vi "send_scenario_config.vi"(0 "simx in":T1={"Config"={"Trajectory"={"Number of frames"=0, "Frame number"=0, "Trajectory"=""}, "Weather"={"id"=""}}, "Connections"={"Simulator Connection"=refnum, "server_ip"="127.0.0.1", "Port"=0, "Sensor connections"=[]}, "Map"={"lanes"={"x"=[], "y"=[], "z"=[]}, "StartPosition"={"start_points"={"locations"=[], "rotations"=[], "type"=[]}, "StartRotation"=[], "StartLocation"=[]}, "Draw Map Size"={"Width"=0, "Height"=0}, "DrawArea"={"min_Y"=0.0, "min_X"=0.0, "Scale X"=0.0, "Scale Y"=0.0}, "Map"=bytes[0], "Map Geojson"=""}}, 2 "Scenario Configuration":path, 5 "error in":errorcluster) -> (6 "simx out":T1={"Config"={"Trajectory"={"Number of frames"=0, "Frame number"=0, "Trajectory"=""}, "Weather"={"id"=""}}, "Connections"={"Simulator Connection"=refnum, "server_ip"="127.0.0.1", "Port"=0, "Sensor connections"=[]}, "Map"={"lanes"={"x"=[], "y"=[], "z"=[]}, "StartPosition"={"start_points"={"locations"=[], "rotations"=[], "type"=[]}, "StartRotation"=[], "StartLocation"=[]}, "Draw Map Size"={"Width"=0, "Height"=0}, "DrawArea"={"min_Y"=0.0, "min_X"=0.0, "Scale X"=0.0, "Scale Y"=0.0}, "Map"=bytes[0], "Map Geojson"=""}}, 7 "Scenario configuration":string, 8 "error out":errorcluster)   [LabVIEW 2025]
doc: "Reads an scenario file (JSON) and sends it to the server."
uses:
  controls/simx_connection.ctl
  controls/config.ctl
  controls/trajectory.ctl
  controls/weather.ctl
  controls/connections.ctl
  controls/start_points.ctl
  <vilib>/Utility/miscctls.llb/LVBoundsTypeDef.ctl
  tools/simx_common.vi
panel:
  in  "Vehicle \nStart Position":i32 min=-1 max=0 step=1
  out "Response":string
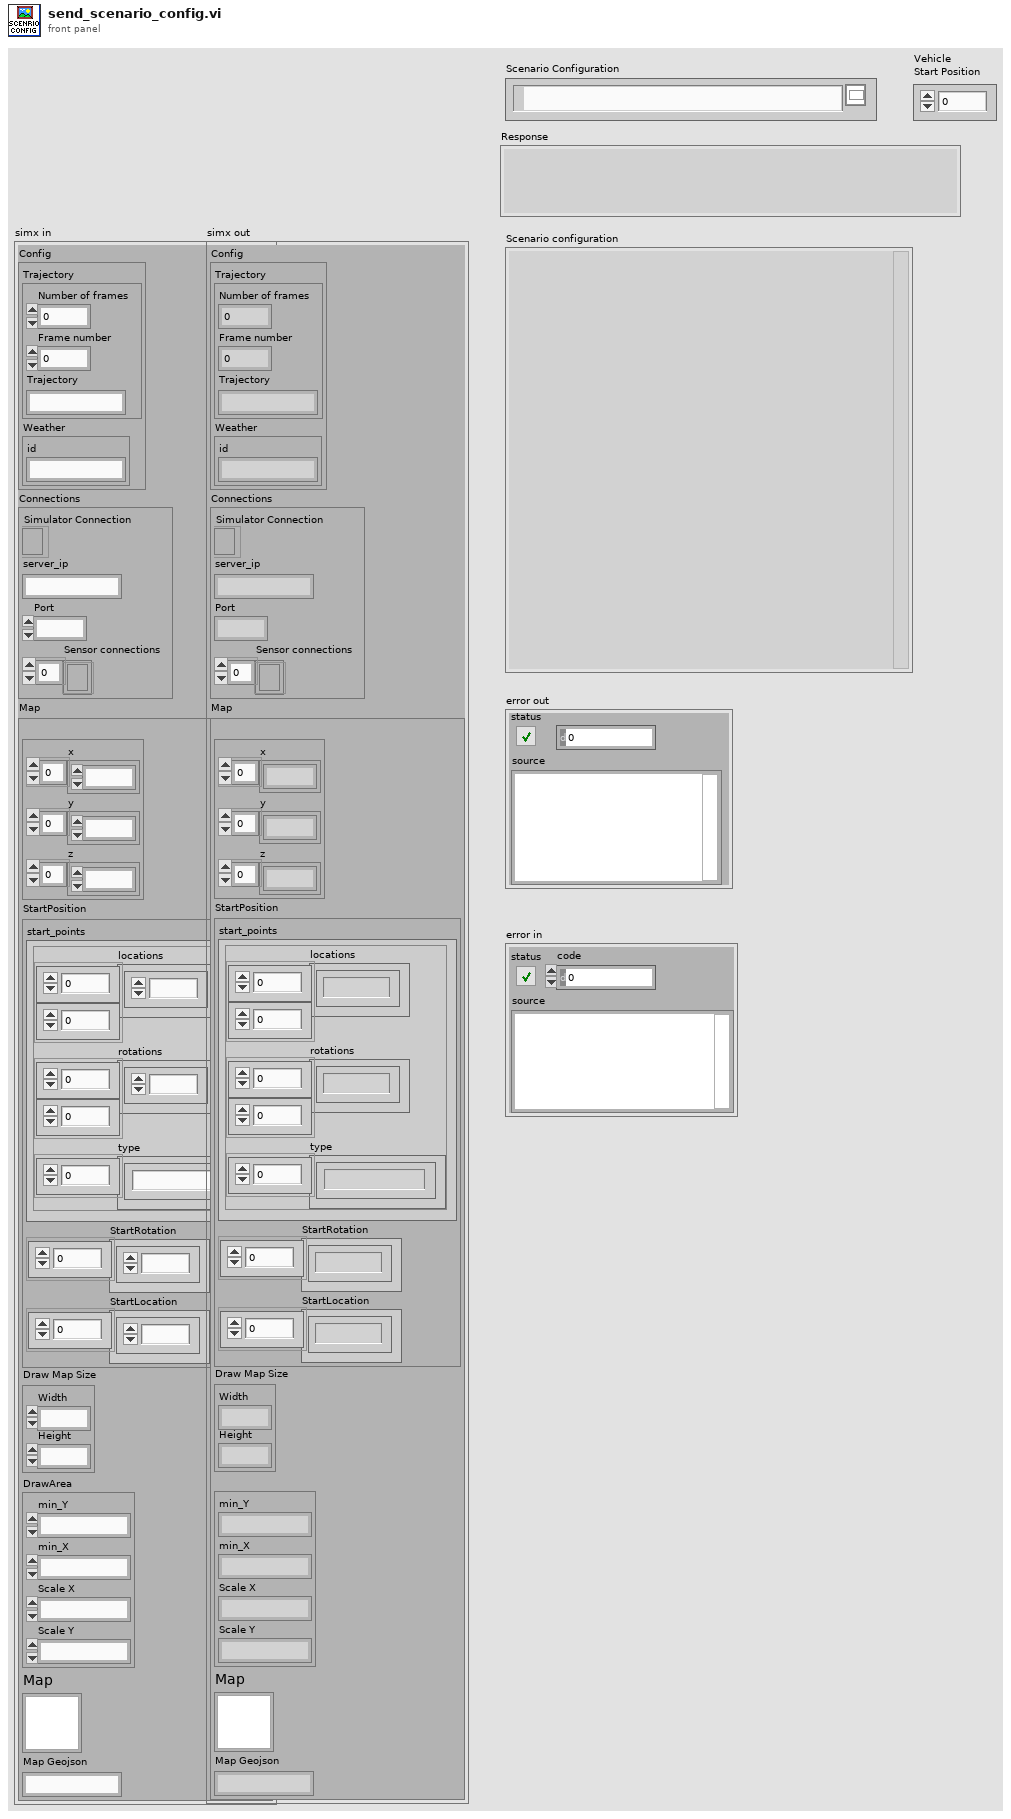
[diagram p1: front panel]
types:
  T1 = typedef "simx_connection.ctl" = cluster{"Config":T2, "Connections":T5, "Map":cluster{"lanes":cluster{"x":dbl[], "y":dbl[], "z":dbl[]}, "StartPosition":cluster{"start_points":T6, "StartRotation":dbl[], "StartLocation":dbl[]}, "Draw Map Size":T7, "DrawArea":cluster{"min_Y":dbl, "min_X":dbl, "Scale X":dbl, "Scale Y":dbl}, "Map":picture, "Map Geojson":string}}
  T2 = typedef "config.ctl" = cluster{"Trajectory":T3, "Weather":T4}
  T3 = typedef "trajectory.ctl" = cluster{"Number of frames":i32, "Frame number":i32, "Trajectory":string}
  T4 = typedef "weather.ctl" = cluster{"id":string}
  T5 = typedef "connections.ctl" = cluster{"Simulator Connection":refnum<k5>, "server_ip":string, "Port":i32, "Sensor connections":refnum<k5>[]}
  T6 = typedef "start_points.ctl" = cluster{"locations":dbl[][], "rotations":dbl[][], "type":string[]}
  T7 = typedef "LVBoundsTypeDef.ctl" = cluster{"Width":u32, "Height":u32}
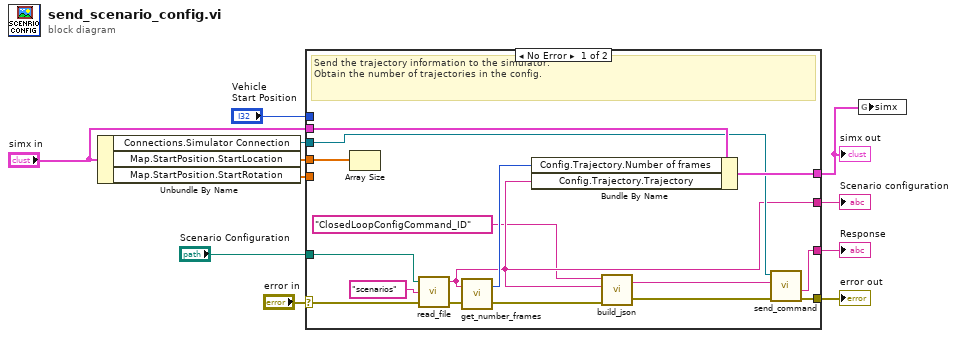
[diagram p0: block diagram]
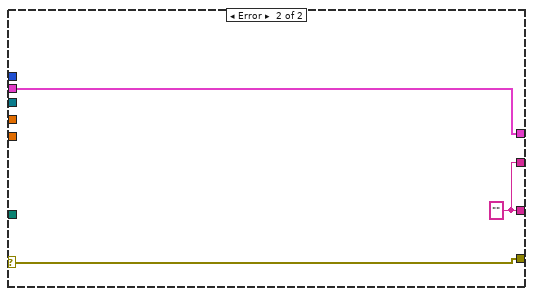
[diagram p2: hidden frame]
diagram:
  n1 = Unbundle By Name("simx in") -> ("Connections.Simulator Connection"=w7:refnum<k5>, "Map.StartPosition.StartLocation"=w4:dbl[], "Map.StartPosition.StartRotation"=w3:dbl[])
  n2 = case shown="No Error" "error in" {
    selector: "error in" -> [w18 w30]
    tunnel: [w27 w28] -> w11
    tunnel: [w26 w30] -> w10
    tunnel: "simx in" -> [w21 w29]
    tunnel: [w22 w29] -> w2
    tunnel: w7 -> [w20 _]
    tunnel: [w14 w28] -> w6
    tunnel: "Scenario Configuration" -> [w15 _]
    tunnel: w4 -> [w17 _]
    tunnel: w3 -> [_ _]
    tunnel: "Vehicle \nStart Position" -> [_ _]
    frame No Error {
      # "Send the trajectory information to the simulator. \nObtain the number of trajectories in the config."
      n3 = Array Size(array=w17) -> ()  [unwired: 1 out]
      n4 = call "read_file.vi"("error in"=w18, "Base directory name"="scenarios" ("Folder path"), "File path in"=w15) -> ("error out"=w19:errorcluster, "Trajectory or Scenario read"=w14:string)  [unwired: 1 out]
      n5 = call "get_number_frames.vi"("error in"=w19, "Trajectory (JSON)"=w14) -> ("error out"=w16:errorcluster, "Number of frames"=w23:i32)
      n6 = Bundle By Name(cluster=w21, "Config.Trajectory.Number of frames"=w23, "Config.Trajectory.Trajectory"=w14) -> (w22:T1)
      n7 = call "build_json.vi"("error in"=w16, "Message"=w14, "Command_ID"="ClosedLoopConfigCommand_ID") -> ("error out"=w24:errorcluster, "JSON Out"=w25:string)  [unwired: 1 in]
      n8 = call "send_command.vi"("error in"=w24, "JSON Command"=w25, "TCP Network Connection in"=w20) -> ("error out"=w26:errorcluster, "Response"=w27:string)  [unwired: 1 in, 2 out]
    }
    frame Error {
      w28 = "" ("response")
    }
  }
  "Response" <- w11
  "error out" <- w10
  "simx out" <- w2
  "Scenario configuration" <- w6
  n9 = global write "simx_common.vi" "simx"(w2) -> ()
